vi "Strategy 1_ works with a lot of noise and fluctuation.vi"() -> ()   [LabVIEW 2018]
doc: "This VI is an example of using the PID VI for a PWM application. For a real application all that is needed is the PID VI and the Output to PWM Logic. Together these can be put in the while loop of a real application.\n\nThis example has defaults tuned to the plant."
uses:
  <vilib>/DAQmx/write.llb/DAQmx Write (Digital 1D Bool 1Chan 1Samp).vi
  <vilib>/DAQmx/create/channels.llb/DAQmx Create Channel (DO-Digital Output).vi
  <vilib>/Waveform/DWDTOps.llb/DWDT Analog to Digital.vi
  <vilib>/Waveform/DWDTOps.llb/DWDT Digital to Boolean Array.vi
  <vilib>/DAQmx/miscellaneous.llb/DAQmx Fill In Error Info.vi
  <vilib>/addons/control/pid/pid.llb/PID (DBL).vi
  <vilib>/addons/control/pid/NI_PID_pid.lvlib
  <vilib>/ptbypt/NI_PtbyPt.lvlib
  <vilib>/measure/NI_MABase.lvlib
panel:
  in  "frequency":dbl=10.0 format="%0.2p"
  out "?":bool
  in  "Exhaust Valve PWM  duty cycle (%)":dbl=50.0
  out "Waveform Chart 2":dbl(graph)
  in  "PID gains":T1={"proportional gain (Kc)"=0.001, "integral time (Ti, min)"=30.0, "derivative time (Td, min)"=0.0} {"derivative time (Td, min)" format="%.3f"; "integral time (Ti, min)" format="%.3f"; "proportional gain (Kc)" format="%.3f"}
  out "PWM Output":bool
  out "Waveform Chart":dbl[][](graph)
  in  "stop":bool
  in  "Setpoint":dbl=500.0 format="%.2f"
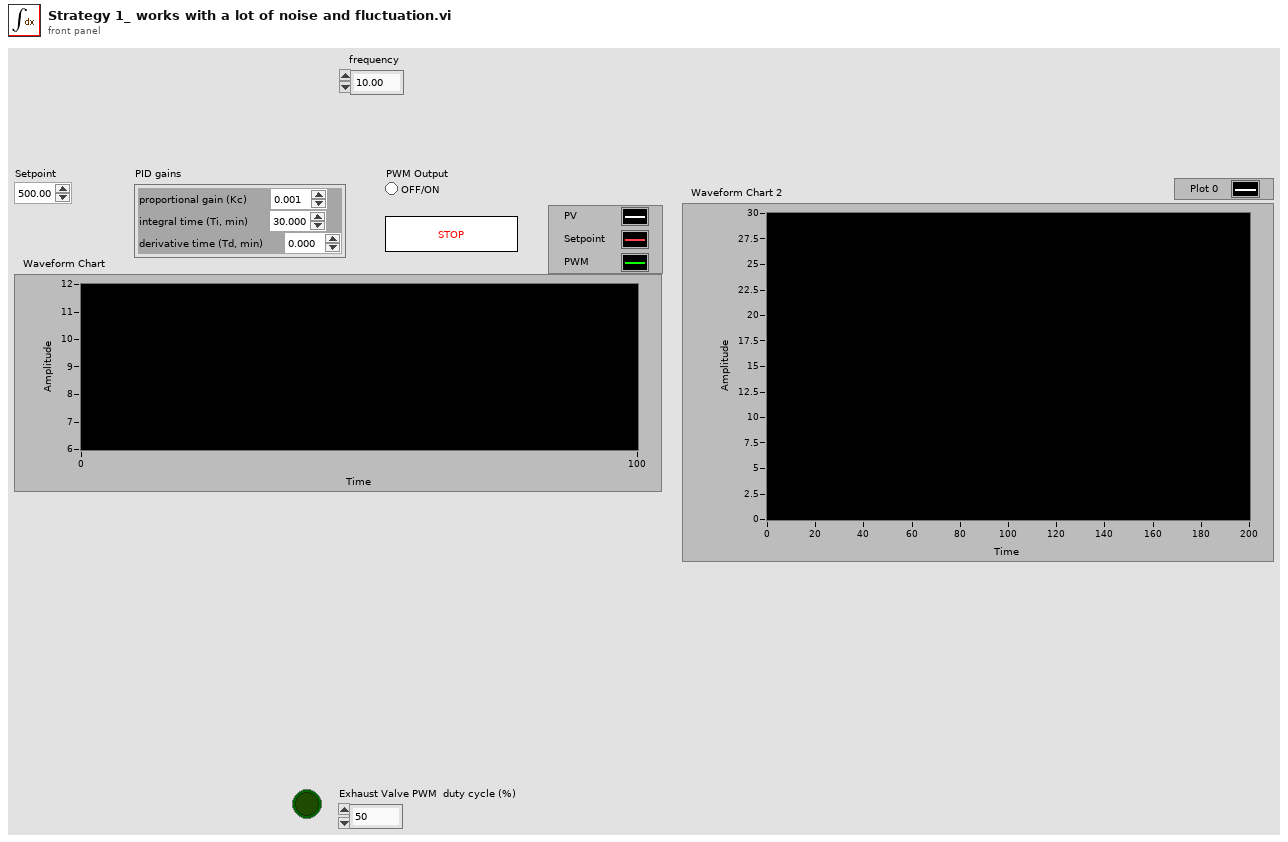
[diagram p1: front panel]
types:
  T1 = cluster{"proportional gain (Kc)":dbl, "integral time (Ti, min)":dbl, "derivative time (Td, min)":dbl}
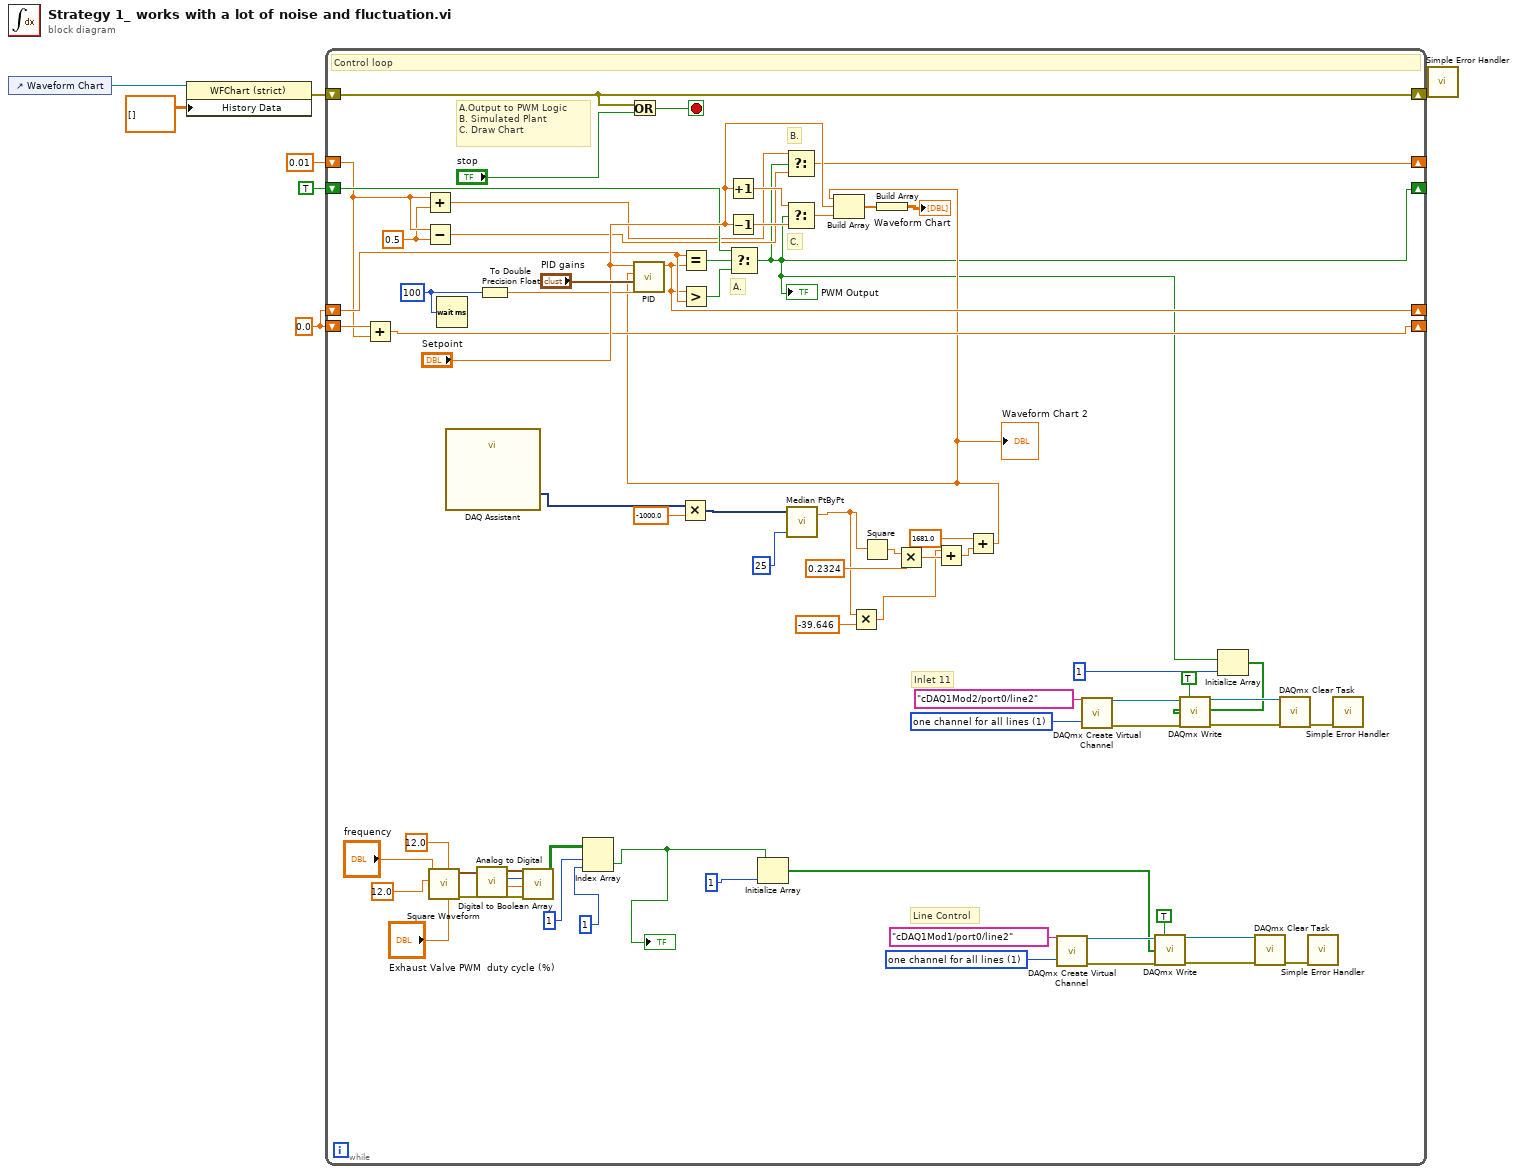
[diagram p0: block diagram]
diagram:
  w6 = 0.0 ("output")
  n1 = control-ref of="Waveform Chart"() -> (w4:refnum<vi>)
  n2 = property class="WFChart (strict)"(reference=w4, "History Data"=dbl[][] []) -> (error out=w3:errorcluster)  [unwired: 1 in, 1 out]
  n3 = while {
    shift-right: [w74] -> _
    shift-left: w6 -> [w75]
    shift-right: [w32] -> _
    shift-left: TRUE -> [w73]
    shift-right: [w71] -> _
    shift-left: w6 -> [w72]
    shift-right: [w69] -> _
    shift-left: 0.01 -> [w70]
    shift-right: [w66] -> w2
    shift-left: w3 -> [w66]
    stop <- w67 stop-if-true
    w25 = 1 items=["one channel for each line", "one channel for all lines"] ("line grouping")
    w45 = 1 items=["one channel for each line", "one channel for all lines"] ("line grouping")
    w58 = 0.5 ("x")
    w77 = u32 100 ("milliseconds to wait")
    # "Line Control"
    # "Inlet 11"
    # "B."
    # "C."
    # "A."
    # "A.Output to PWM Logic \nB. Simulated Plant\nC. Draw Chart"
    # "Control loop"
    n4 = Add(x=w72, y=w70) -> (x+y=w71:dbl)
    n5 = Add(x=w70, y=w58) -> (x+y=w59:dbl)
    n6 = Subtract(x=w70, y=w58) -> (x-y=w57:dbl)
    n7 = call <vilib>:"Square Waveform.vi"("duty cycle (%)"="Exhaust Valve PWM  duty cycle (%)", "offset"=12.0, "amplitude"=12.0, "frequency"="frequency") -> ("error out"=w17:errorcluster, "signal out"=w11:waveform(dbl))  [unwired: 6 in]
    n8 = Wait (ms)(milliseconds to wait=w77) -> ()  [unwired: 1 out]
    n9 = call "DAQ Assistant"() -> ("data"=w55:dynamicdata)  [unwired: 17 in, 2 out]
    n10 = call-poly <vilib>:"Analog to Digital.vi"("error in (no error)"=w17, "analog waveform"=w11) -> ("error out"=w19:errorcluster, "full-scale range (out)"=w20:dbl, "resolution (out)"=w21:i32, "digital waveform"=w18:digitalwaveform)  [unwired: 6 in]
    n11 = To Double Precision Float(number=w77) -> (double precision float=w56:dbl)
    n12 = call-poly <vilib>:"Digital to Boolean Array.vi"("error in (no error)"=w19, "mode"=w20, "response on error"=w21, "digital waveform"=w18) -> ("boolean array"=w23:bool[][])  [unwired: 6 in, 1 out]
    n13 = Index Array(array=w23, index (row)=1, index (col)=1 ("disabled index (col)")) -> (element=w10:bool)
    "?" <- w10
    n14 = Or(x=w66, y="stop") -> (x .or. y?=w67:bool)
    n15 = Multiply(x=w55, y=-1000.0) -> (x*y=w53:dynamicdata)
    n16 = Increment(x="Setpoint") -> (x+1=w63:dbl)
    n17 = Decrement(x="Setpoint") -> (x-1=w62:dbl)
    n18 = Initialize Array(w10, 1 ("dimension size")) -> (w9:bool[])
    n19 = call <vilib>:"Median PtByPt.vi"("sample length"=25, "x"=w53) -> ("median"=w39:dbl)  [unwired: 2 in, 1 out]
    n20 = Multiply(x=w39, y=-39.646) -> (x*y=w36:dbl)
    n21 = Square(x=w39) -> (x^2=w41:dbl)
    n22 = Multiply(x=w41, y=0.2324) -> (x*y=w37:dbl)
    n23 = Add(x=w36, y=w37) -> (x+y=w35:dbl)
    n24 = Add(x=1681.0, y=w35) -> (x+y=w33:dbl)
    "Waveform Chart 2" <- w33
    n25 = call-poly <vilib>:"PID.vi"("dt (s)"=w56, "PID gains"="PID gains", "process variable"=w33, "setpoint"="Setpoint") -> ("output"=w74:dbl)  [unwired: 6 in, 1 out]
    n26 = Equal?(x=w75, y=w74) -> (x = y?=w65:bool)
    n27 = Greater?(x=w74, y=w75) -> (0:w64:bool)
    n28 = Select(t=w73, s=w65, f=w64) -> (s? t:f=w32:bool)
    "PWM Output" <- w32
    n29 = Select(t=w59, s=w32, f=w57) -> (s? t:f=w69:dbl)
    n30 = Select(t=w63, s=w32, f=w62) -> (s? t:f=w61:dbl)
    n31 = Build Array(w33, "Setpoint", w61) -> (w60:dbl[])
    n32 = Build Array(w60) -> (→"Waveform Chart":dbl[][])
    n33 = call-poly <vilib>:"DAQmx Create Virtual Channel.vi"("lines"=tag "cDAQ1Mod1/port0/line2", "line grouping"=w25) -> ("task out"=w27:refnum<k21>, "error out"=w26:errorcluster)  [unwired: 12 in]
    n34 = call-poly <vilib>:"DAQmx Create Virtual Channel.vi"("lines"=tag "cDAQ1Mod2/port0/line2", "line grouping"=w45) -> ("task out"=w47:refnum<k21>, "error out"=w46:errorcluster)  [unwired: 12 in]
    n35 = call-poly <vilib>:"DAQmx Write.vi"("task/channels in"=w27, "auto start"=TRUE, "data"=w9, "error in"=w26) -> ("task out"=w29:refnum<k21>, "error out"=w30:errorcluster)  [unwired: 9 in, 1 out]
    n36 = Initialize Array(w32, 1 ("dimension size")) -> (w42:bool[])
    n37 = call-poly <vilib>:"DAQmx Write.vi"("task/channels in"=w47, "auto start"=TRUE, "data"=w42, "error in"=w46) -> ("task out"=w49:refnum<k21>, "error out"=w50:errorcluster)  [unwired: 9 in, 1 out]
    n38 = call <vilib>:"DAQmx Clear Task.vi"("task in"=w29, "error in"=w30) -> ("error out"=w24:errorcluster)  [unwired: 13 in]
    n39 = call <vilib>:"DAQmx Clear Task.vi"("task in"=w49, "error in"=w50) -> ("error out"=w44:errorcluster)  [unwired: 13 in]
    n40 = call <vilib>:"Simple Error Handler.vi"("error in (no error)"=w24) -> ()  [unwired: 4 in, 5 out]
    n41 = call <vilib>:"Simple Error Handler.vi"("error in (no error)"=w44) -> ()  [unwired: 4 in, 5 out]
  }
  n42 = call <vilib>:"Simple Error Handler.vi"("error in (no error)"=w2) -> ()  [unwired: 4 in, 5 out]
